vi "Handle Command.vi"(8 "error in (no error)":errorcluster, 9 "Data":variant, 10 "Command":string, 11 "instrument.Cryostation in":refnum<class "instrument.Cryostation.lvclass">) -> (0 "error out":errorcluster, 1 "Processed Data":variant, 2 "Command":string, 3 "instrument.Cryostation out":refnum<class "instrument.Cryostation.lvclass">)   [LabVIEW 2019, in "instrument.Cryostation.lvclass"]
uses:
  instrument.Cryostation.lvclass
  <userlib>/LevyLab/Instrument Framework/Instrument Types/Cryostat/Typedefs/getTemperature--cluster.ctl
  instrument.Cryostation.lvclass/instrument.Cryostation.ctl
  c23db690-3157-4935-b6ba-6af88c6a11b9.vi
  c23db690-3157-4935-b6ba-6af88c6a11b9.vi/93065efb-0245-4967-af1b-a07a0eba3ab9.vi
  c23db690-3157-4935-b6ba-6af88c6a11b9.vi/d57035eb-8c83-4ecf-8fff-8779856d9edb.vi
  <vilib>/Utility/Data Type/Get Type Information.vi
  <vilib>/JDP Science/JSONtext/JSON text to Variant.vi
  <vilib>/JDP Science/JSONtext/LVClass Serializer/JSONtext LVClass Serializer.lvclass
  <userlib>/LevyLab/Instrument Framework/Instrument Types/Cryostat/Instrument.Cryostat.lvclass
  58c8ddcc-542a-4dc2-9390-b04d59754b4b.vi
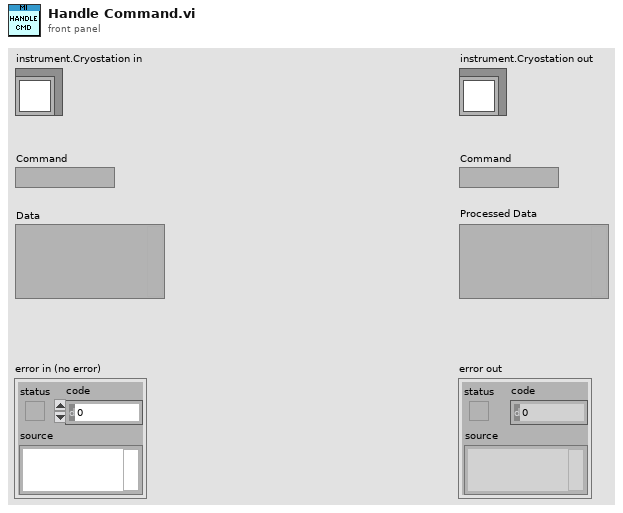
[diagram p1: front panel]
types:
  T1 = typedef "Instrument.Cryostat.lvclass/getTemperature--cluster.ctl" = cluster{"temperature":dbl, "status":string, "finished":bool}
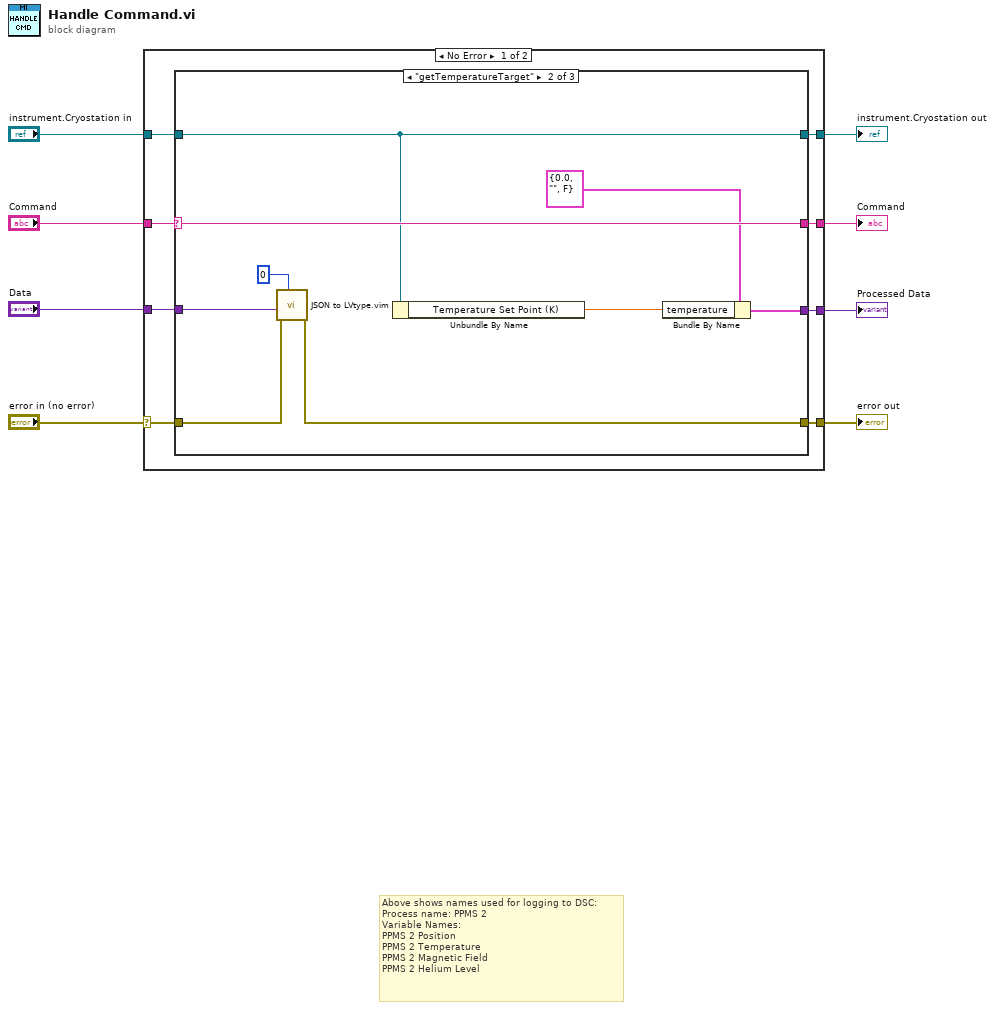
[diagram p0: block diagram]
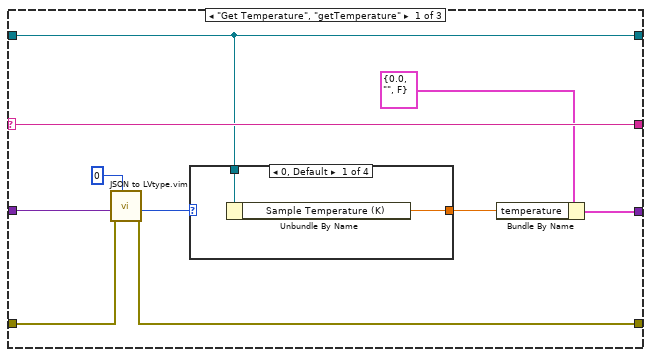
[diagram p2: hidden frame]
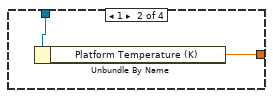
[diagram p3: hidden frame]
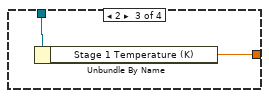
[diagram p4: hidden frame]
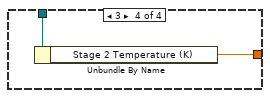
[diagram p5: hidden frame]
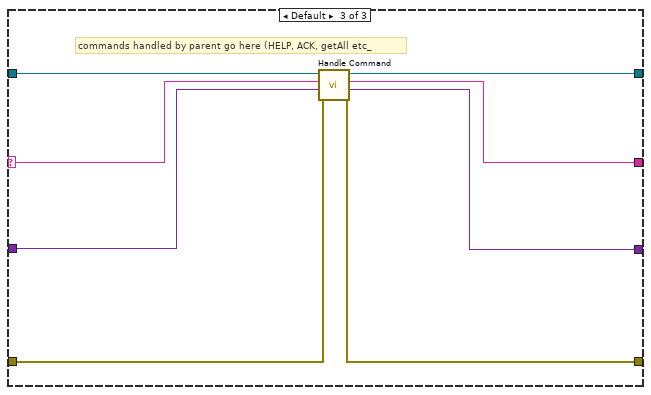
[diagram p6: hidden frame]
diagram:
  # "Above shows names used for logging to DSC:\nProcess name: PPMS 2\nVariable Names:\nPPMS 2 Position\nPPMS 2 Temperature\nPPMS 2 Magnetic Field\nPPMS 2 Helium Level"
  n1 = case shown="No Error" "error in (no error)" {
    selector: "error in (no error)" -> [w11 w52]
    tunnel: [w10 w52] -> w6
    tunnel: [w16 _] -> w4
    tunnel: [w15 _] -> w5
    tunnel: [w14 w53] -> w7
    tunnel: "Data" -> [w13 _]
    tunnel: "Command" -> [w9 _]
    tunnel: "instrument.Cryostation in" -> [w12 w53]
    frame No Error {
      n2 = case shown="\"getTemperatureTarget\"" w9 {
        selector: w9 -> [w21 w39 w46]
        tunnel: [w19 w37 w44] -> w16
        tunnel: [w21 w39 w51] -> w15
        tunnel: [w17 w35 w50] -> w14
        tunnel: w13 -> [w23 w41 w45]
        tunnel: w12 -> [w17 w35 w49]
        tunnel: w11 -> [w26 w43 w48]
        tunnel: [w25 w42 w47] -> w10
        frame "Get Temperature", "getTemperature" {
          n3 = call "JSON to LVtype.vim"("type"=0 ("Channel"), "error in (no error)"=w26, "JSON Data in"=w23) -> ("error out"=w25:errorcluster, "Data out"=w24:i32)  [unwired: 7 in]
          n4 = case shown="0, Default" w24 {
            tunnel: [w28 w30 w32 w34] -> w18
            tunnel: w17 -> [w27 w29 w31 w33]
            frame 0, Default {
              n5 = Unbundle By Name(w27) -> ("Sample Temperature (K)"=w28:dbl)
            }
            frame 1 {
              n6 = Unbundle By Name(w29) -> ("Platform Temperature (K)"=w30:dbl)
            }
            frame 2 {
              n7 = Unbundle By Name(w31) -> ("Stage 1 Temperature (K)"=w32:dbl)
            }
            frame 3 {
              n8 = Unbundle By Name(w33) -> ("Stage 2 Temperature (K)"=w34:dbl)
            }
          }
          n9 = Bundle By Name(cluster=T1 {"temperature"=0.0, "status"="", "finished"=FALSE} ("getTemperature"), "temperature"=w18) -> (w19:T1)
        }
        frame "getTemperatureTarget" {
          n10 = call "JSON to LVtype.vim"("type"=0 ("Channel"), "error in (no error)"=w43, "JSON Data in"=w41) -> ("error out"=w42:errorcluster)  [unwired: 7 in, 1 out]
          n11 = Unbundle By Name(w35) -> ("Temperature Set Point (K)"=w36:dbl)
          n12 = Bundle By Name(cluster=T1 {"temperature"=0.0, "status"="", "finished"=FALSE} ("getTemperature"), "temperature"=w36) -> (w37:T1)
        }
        frame Default {
          # "commands handled by parent go here (HELP, ACK, getAll etc_"
          n13 = call-parent "Handle Command.vi"("error in (no error)"=w48, "params in"=w45, "command"=w46, "Instrument in"=w49) -> ("error out"=w47:errorcluster, "processed data"=w44:variant, "command out"=w51:string, "Instrument out"=w50:refnum<class "instrument.Cryostation.lvclass">)  [unwired: 4 in]
        }
      }
    }
    frame Error {
    }
  }
  "error out" <- w6
  "instrument.Cryostation out" <- w7
  "Processed Data" <- w4
  "Command" <- w5
